vi "GetNotifier.vi"(8 "error in (no error)":errorcluster, 11 "ClassByRef in":refnum<class "ClassByRef.lvclass">) -> (0 "error out":errorcluster, 2 "notifier":refnum<notifier>, 3 "ClassByRef out":refnum<class "ClassByRef.lvclass">)   [LabVIEW 2021, in "ClassUtilities.lvlib" / "ClassByRef.lvclass"]
uses:
  ClassByRef.lvclass
  ClassByRef.lvclass/ClassByRef.ctl
  815770e3-f244-4544-877a-43bf45f14863.vi
  GetRef.vi
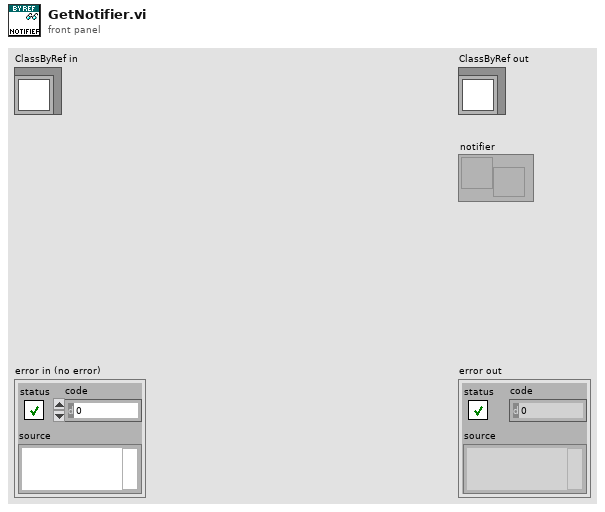
[diagram p1: front panel]
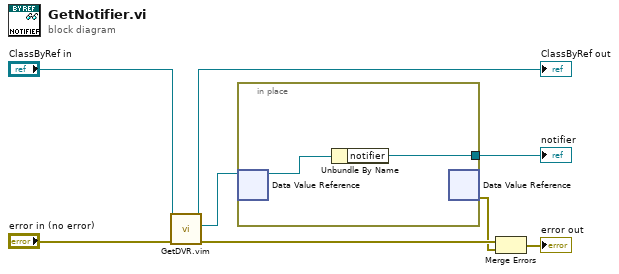
[diagram p0: block diagram]
diagram:
  n1 = call "GetDVR.vim"("error in (no error)"="error in (no error)", "ByRefClass in"="ClassByRef in") -> ("error out"=w7:errorcluster, "DVR"=w3:refnum<data-value>, "ByRefClass out"=→"ClassByRef out":refnum<class "ClassByRef.lvclass">)  [unwired: 7 in]
  n2 = in-place {
    in-place-border: [w9] -> w4
    n3 = in-place-dvr #1(w3) -> (w10:refnum<class "ClassByRef.lvclass">)  [unwired: 1 out]
    n4 = Unbundle By Name(w10) -> ("notifier"=w9:refnum<notifier>)
    n5 = in-place-dvr #1() -> (w1:errorcluster)  [unwired: 1 in, 1 out]
  }
  "notifier" <- w4
  n6 = Merge Errors(w7, w1) -> (→"error out":errorcluster)
